vi "WILT Find Agilent Station Headers.vi"(11 "Full Agilent Array":T1) -> (3 "Data Out Array":T1)   [LabVIEW 2016]
uses:
  Type Definitions/WILT Agilent Data Cluster.ctl
  Type Definitions/WILT Agilent Channel Definition.ctl
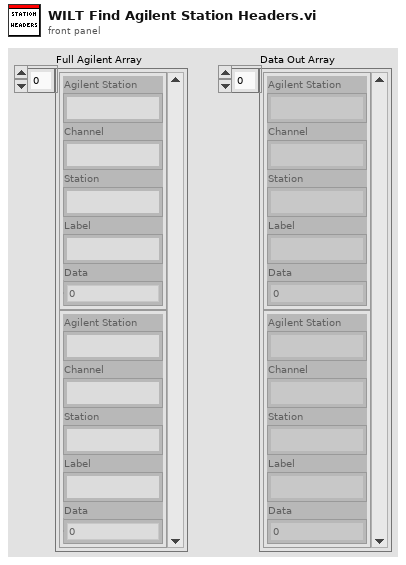
[diagram p1: front panel]
types:
  T1 = typedef "WILT Agilent Data Cluster.ctl" = T2[]
  T2 = typedef "WILT Agilent Channel Definition.ctl" = cluster{"Channel":string, "Station":string, "Label":string, "Agilent Station":string, "Data":dbl}
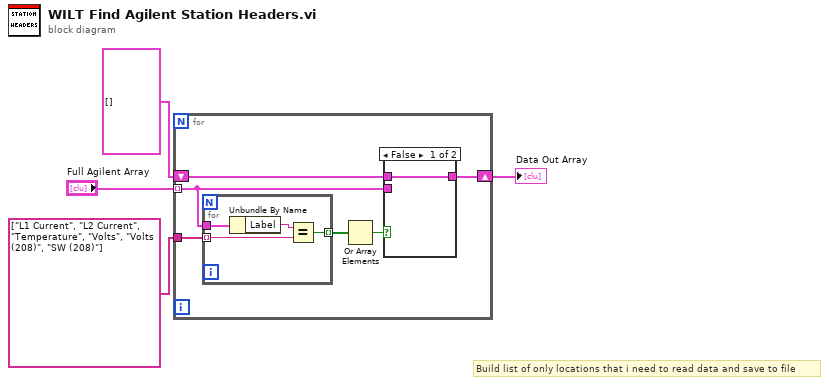
[diagram p0: block diagram]
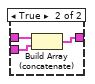
[diagram p2: hidden frame]
diagram:
  # "Build list of only locations that i need to read data and save to file"
  n1 = for {
    tunnel: "Full Agilent Array" -> [w6] mode=indexing
    tunnel: string[] ["L1 Current", "L2 Current", "Temperature", "Volts", "Volts (208)", "SW (208)"] -> [w10]
    shift-right: [w5] -> w3
    shift-left: T1 [] ("Data IN Array") -> [w7]
    n2 = for {
      tunnel: w6 -> [w18]
      tunnel: w10 -> [w16] mode=indexing
      tunnel: [w15] -> w9 mode=indexing
      n3 = Unbundle By Name(w18) -> ("Label"=w17:string)
      n4 = Equal?(x=w17, y=w16) -> (x = y?=w15:bool)
    }
    n5 = Or Array Elements(Boolean array=w9) -> (logical OR=w8:bool)
    n6 = case shown="False" w8 {
      tunnel: w7 -> [w11 w14]
      tunnel: w6 -> [_ w12]
      tunnel: [w11 w13] -> w5
      frame False {
      }
      frame True {
        n7 = Build Array (concatenate)(w14, w12) -> (w13:T1)
      }
    }
  }
  "Data Out Array" <- w3
